vi "State_Machine.vi"(8 "error in (no error)":errorcluster caption="entrée d'erreur (pas d'erreur)", 11 "Get_Voltage en entrée":refnum<class "Zigbee_Set_Manufacturer_id.lvclass">) -> (0 "error out":errorcluster caption="sortie d'erreur", 2 "Json_String":string, 3 "Get_Voltage en sortie":refnum<class "Zigbee_Set_Manufacturer_id.lvclass">)   [LabVIEW 2020, in "Library Test.lvlib" / "Zigbee_Set_Manufacturer_id.lvclass"]
uses:
  Zigbee_Set_Manufacturer_id.lvclass
  C:/Users/ngarcin/OneDrive - Altyor/Standard TB/Class/Test/Test (Default)/Test (Default).lvclass
  C:/Users/ngarcin/OneDrive - Altyor/Standard TB/Class/Test/Zigbee_Send_Command_UART/Zigbee_Send_Command_UART.lvclass
  JSON API/JSON Value/Set from JSON string.vi
  JSON API/JSON Value/JSON Value.lvclass
  Zigbee_Send_Command_UART/Zigbee_Send_Command_UART.lvclass
  Zigbee_Set_Manufacturer_id.lvclass/Zigbee_Set_Manufacturer_id.ctl
  JSON API/Variant JSON/Variant JSON.lvlib
  JSON API/Get Polymorphic/JSON GetSet.lvlib
  Commun VI/Library Commun.lvlib
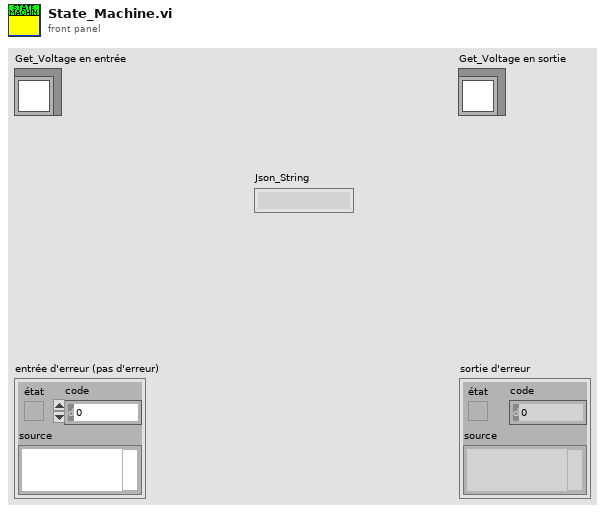
[diagram p1: front panel]
types:
  T1 = enum16{"Get Variable", "Get All Variables", "Set Variable", "Delete Variable", "Delete All Variable"}
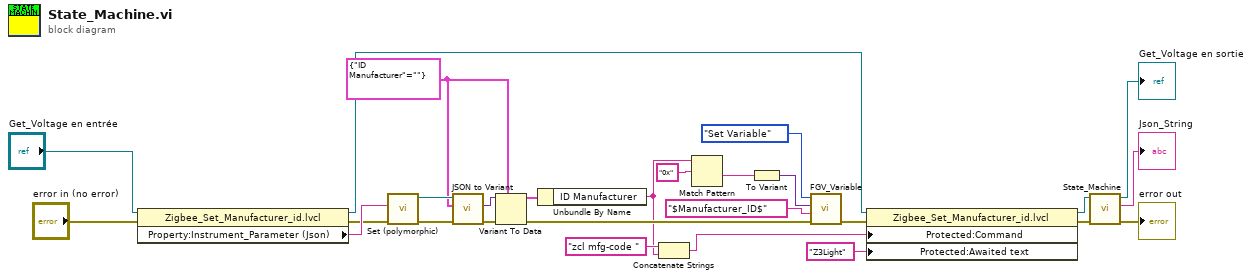
[diagram p0: block diagram]
diagram:
  w18 = cluster{"ID Manufacturer":string} {"ID Manufacturer"=""}
  n1 = property class="Zigbee_Set_Manufacturer_id.lvcl"(reference="Get_Voltage en entrée", error in="error in (no error)") -> (reference out=w17:refnum<class "Zigbee_Set_Manufacturer_id.lvclass">, error out=w19:errorcluster, "Property:Instrument_Parameter (Json)"=w20:string)
  n2 = call-poly "Set (polymorphic).vi"("error in (no error)"=w19, "JSON stream"=w20) -> ("error out"=w22:errorcluster, "JSON Value out"=w24:refnum<class "JSON Value.lvclass">)  [unwired: 7 in, 1 out]
  n3 = call "JSON to Variant.vi"("error in (no error)"=w22, "Variant (Data Type)"=w18, "JSON Value"=w24) -> ("error out"=w23:errorcluster, "Variant out"=w21:variant)  [unwired: 7 in]
  n4 = Variant To Data(error in=w23, type=w18, Variant=w21) -> (data=w16:cluster{"ID Manufacturer":string}, error out=w6:errorcluster)
  n5 = Unbundle By Name(w16) -> ("ID Manufacturer"=w3:string)
  n6 = Concatenate Strings("zcl mfg-code " ("Command"), w3) -> (w14:string)
  n7 = Match Pattern(string=w3, regular expression="0x" ("expression régulière")) -> (after substring=w4:string)  [unwired: 1 in, 3 out]
  n8 = To Variant(anything=w4) -> (Variant=w7:variant)
  n9 = call "FGV_Variable.vi"("error in (no error)"=w6, "Variable"="$Manufacturer_ID$" ("Variable Printable"), "Data In"=w7, "Function"=T1."Set Variable") -> ("error out"=w5:errorcluster)  [unwired: 5 in, 2 out]
  n10 = property class="Zigbee_Set_Manufacturer_id.lvcl"(reference=w17, error in=w5, "Protected:Command"=w14, "Protected:Awaited text"="Z3Light" ("Awaited text")) -> (reference out=w11:refnum<class "Zigbee_Set_Manufacturer_id.lvclass">, error out=w10:errorcluster)
  n11 = call-parent "State_Machine.vi"("error in (no error)"=w10, "Send_Frame en entrée"=w11) -> ("error out"=→"error out":errorcluster, "Json_String"=→"Json_String":string, "Send_Frame en sortie"=→"Get_Voltage en sortie":refnum<class "Zigbee_Set_Manufacturer_id.lvclass">)  [unwired: 7 in]
